vi "TSP-Link Set Node Number.vi"(7 "Node Number (1)":i32=1 min=1 max=64, 8 "error in (no error)":errorcluster, 11 "VISA resource name":refnum<visa-resource-name>) -> (0 "error out":errorcluster, 3 "VISA resource name out":refnum<visa-resource-name>, 4 "Command String":string)   [LabVIEW 2009, in "Keithley 2600 Series.lvlib"]
doc: "This VI sets the connected instrument's TSP-Link node number.\n\n<b>Functions and Attributes Used</b>\ntsplink.node\n\nNote:\nTSP-Link feature is not supported with Keithley 2604B, 2614B, 2634B."
uses:
  <instrlib>/Keithley 2600 Series/Keithley 2600 Series.lvlib
  <instrlib>/Keithley 2600 Series/Private/GlobalVariables.vi
panel:
  # "(c) 2008 Keithley Instruments, Inc.  ALL RIGHTS RESERVED."
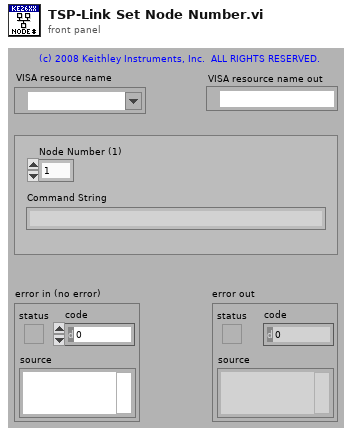
[diagram p1: front panel]
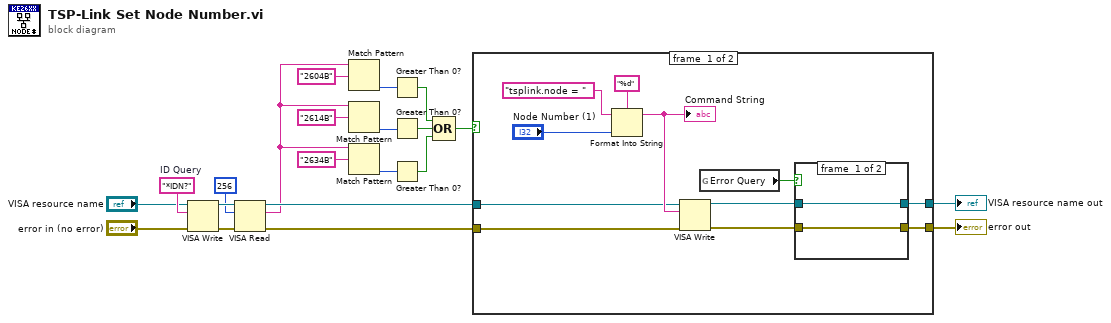
[diagram p0: block diagram]
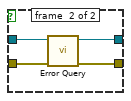
[diagram p2: hidden frame]
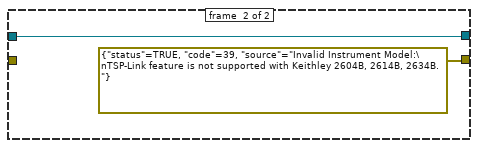
[diagram p3: hidden frame]
diagram:
  w16 = "*IDN?"  # ID Query
  n1 = VISA Write(VISA resource name="VISA resource name", write buffer=w16, error in (no error)="error in (no error)") -> (VISA resource name out=w19:refnum<visa-resource-name>, error out=w18:errorcluster)  [unwired: 1 out]
  n2 = VISA Read(VISA resource name=w19, byte count=u32 256, error in (no error)=w18) -> (VISA resource name out=w13:refnum<visa-resource-name>, read buffer=w1:string, error out=w12:errorcluster)  [unwired: 1 out]
  n3 = Match Pattern(string=w1, regular expression="2604B" ("y")) -> (offset past match=w8:i32)  [unwired: 1 in, 3 out]
  n4 = Match Pattern(string=w1, regular expression="2614B" ("y")) -> (offset past match=w7:i32)  [unwired: 1 in, 3 out]
  n5 = Match Pattern(string=w1, regular expression="2634B" ("y")) -> (offset past match=w6:i32)  [unwired: 1 in, 3 out]
  n6 = Greater Than 0?(x=w8) -> (x > 0?=w5:bool)
  n7 = Greater Than 0?(x=w7) -> (x > 0?=w4:bool)
  n8 = Greater Than 0?(x=w6) -> (x > 0?=w3:bool)
  n9 = Compound Arithmetic op=OR(w5, w4, w3) -> (w2:bool)
  n10 = case shown="False" w2 {
    tunnel: [w25 w40] -> w21
    tunnel: [w24 errorcluster {"status"=TRUE, "code"=39, "source"="Invalid Instrument Model:\nTSP-Link feature is not supported with Keithley 2604B, 2614B, 2634B."} ("error out")] -> w20
    tunnel: w13 -> [w23 w40]
    tunnel: w12 -> [w22 _]
    frame #0 {
      n11 = Format Into String(format string="%d", initial string="tsplink.node = " ("command"), "Node Number (1)") -> (resulting string=w29:string)  [unwired: 1 in, 1 out]
      "Command String" <- w29
      n12 = VISA Write(VISA resource name=w23, write buffer=w29, error in (no error)=w22) -> (VISA resource name out=w27:refnum<visa-resource-name>, error out=w26:errorcluster)  [unwired: 1 out]
      n13 = global read "GlobalVariables.vi" "Error Query"() -> (w28:bool)
      n14 = case shown="True" w28 {
        tunnel: w27 -> [w34 w38]
        tunnel: w26 -> [w33 w37]
        tunnel: [w34 w36] -> w25
        tunnel: [w33 w35] -> w24
        frame #0 {
        }
        frame #1 {
          n15 = call <instrlib>:"Error Query.vi"("error in (no error)"=w37, "VISA resource name"=w38) -> ("error out"=w35:errorcluster, "VISA resource name out"=w36:refnum<visa-resource-name>)  [unwired: 8 out]
        }
      }
    }
    frame #1 {
    }
  }
  "VISA resource name out" <- w21
  "error out" <- w20
